vi "Destroy Texture.vi"(8 "error in":errorcluster, 11 "Texture Pointer":u32 format="%.0x") -> (0 "error out":errorcluster)   [LabVIEW 2015, in "LibSDL2.lvlib"]
uses:
  LibSDL2.lvlib
  DLL/SDL2.dll
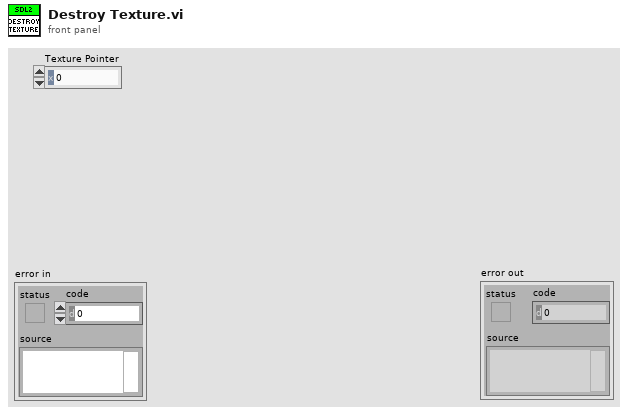
[diagram p1: front panel]
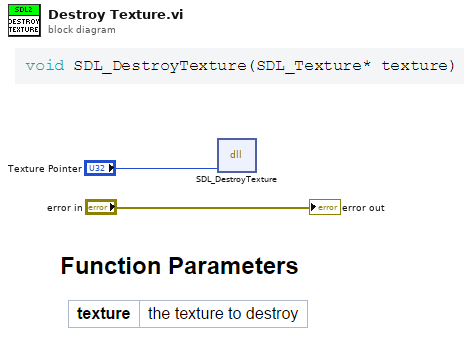
[diagram p0: block diagram]
diagram:
  n1 = dll-call lib="C:/dev/PGS/LabSDL2/Source/Libraries/LibSDL2 Wrapper/DLL/SDL2.dll" fn="SDL_DestroyTexture"("texture"="Texture Pointer") -> ()  [unwired: 5 in, 2 out]
  "error out" <- "error in"
